vi "Write States.vi"(8 "error in (no error)":errorcluster, 10 "States 2":T1(ring), 11 "PenaltyTactic in":refnum<class "PenaltyTactic.lvclass">) -> (0 "error out":errorcluster, 3 "PenaltyTactic out":refnum<class "PenaltyTactic.lvclass">)   [LabVIEW 2023, in "PenaltyTactic.lvclass"]
uses:
  PenaltyTactic.lvclass
  PenaltyTactic.lvclass/PenaltyTactic.ctl
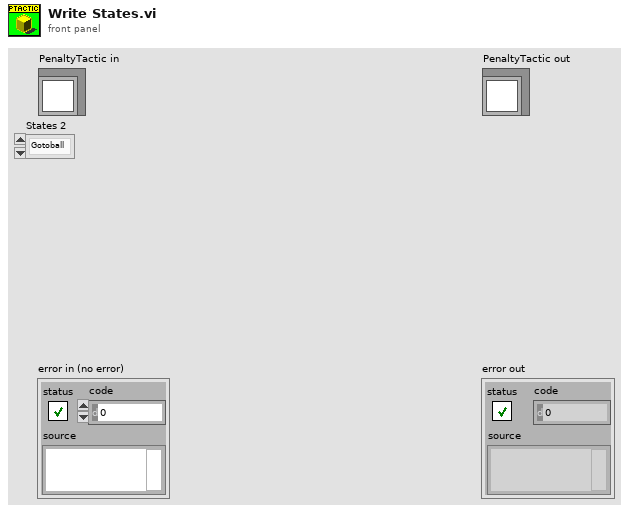
[diagram p1: front panel]
types:
  T1 = enum16{"Gotoball", "Kick", "Fake kick", "Position", "Exit"}
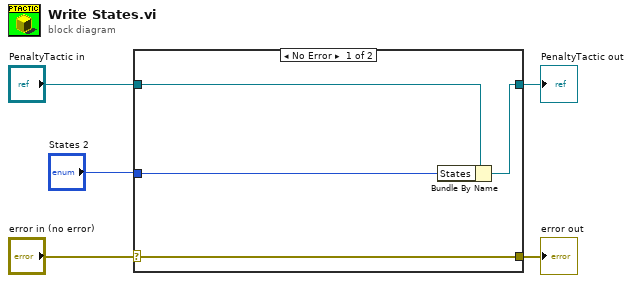
[diagram p0: block diagram]
diagram:
  n1 = case shown="No Error" "error in (no error)" {
    selector: "error in (no error)" -> [w9 w10]
    tunnel: [w9 w10] -> w4
    tunnel: [w7 w11] -> w2
    tunnel: "PenaltyTactic in" -> [w8 w11]
    tunnel: "States 2" -> [w6 _]
    frame No Error {
      n2 = Bundle By Name(cluster=w8, "States"=w6) -> (w7:refnum<class "PenaltyTactic.lvclass">)
    }
    frame Error {
    }
  }
  "error out" <- w4
  "PenaltyTactic out" <- w2
